vi "Pendant, show poses.vi"() -> (1 "position":string, 3 "group":string)   [LabVIEW 2013]
uses:
  <vilib>/Utility/config.llb/NI_LVConfig.lvlib
panel:
  in  "tab":T1(tab)
  in  "Groups":i32(listbox)
  in  "position":i32(listbox)
  in  "continue":bool
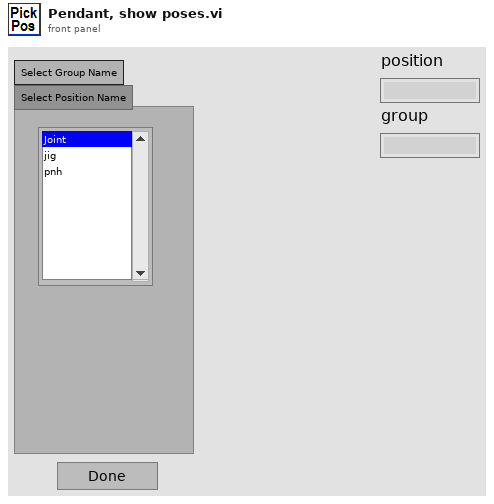
[diagram p1: front panel]
types:
  T1 = enum32{"Select Group Name", "Select Position Name"}
  T2 = typedef "NI_LVConfig.lvlib/Config Data RefNum.ctl" = refnum<k1>
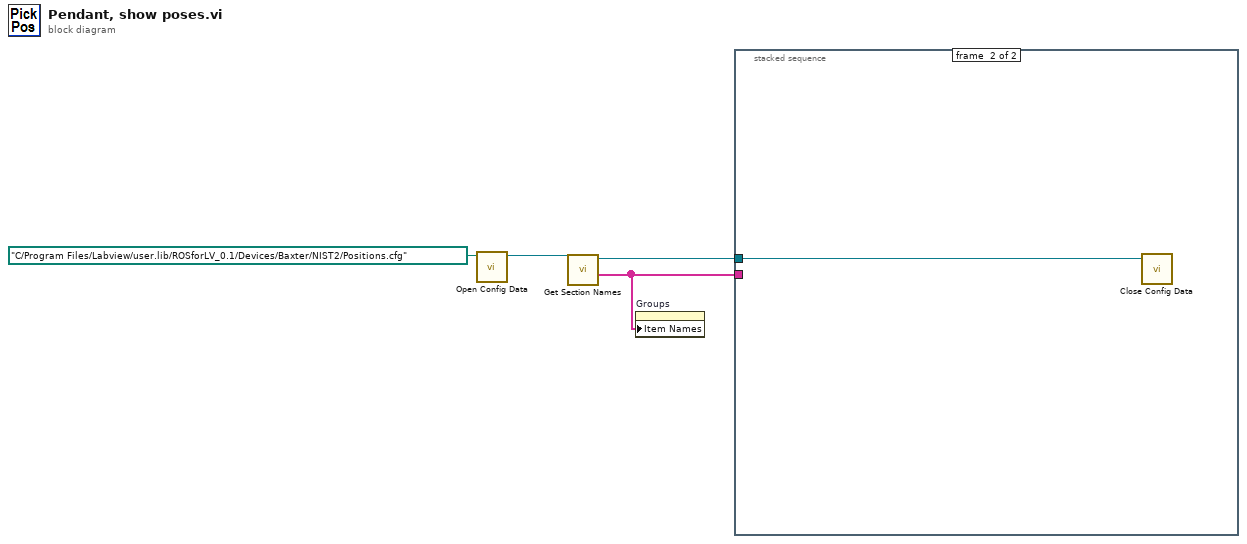
[diagram p0: block diagram]
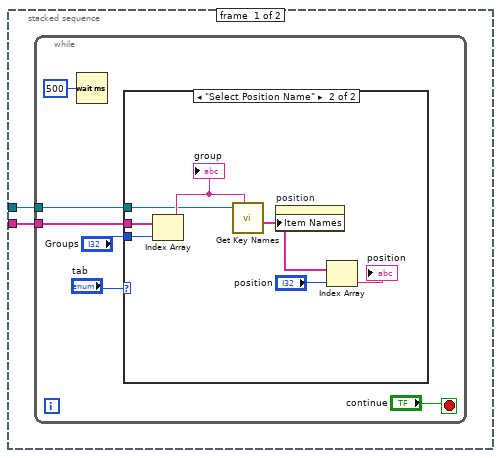
[diagram p2: hidden frame]
diagram:
  n1 = call <vilib>:"Open Config Data.vi"("configuration file path"=path "C:/Program Files/Labview/user.lib/ROSforLV_0.1/Devices/Baxter/NIST2/Positions.cfg") -> ("refnum"=w3:T2)  [unwired: 8 in, 2 out]
  n2 = call <vilib>:"Get Section Names.vi"("refnum"=w3) -> ("section names"=w2:string[], "refnum out"=w1:T2)  [unwired: 8 in, 1 out]
  n3 = property on="Groups" class="LstBox (strict)"("Item Names"=w2) -> ()  [unwired: 2 in, 2 out]
  n4 = stacked-sequence {
    tunnel: w2 -> [w6 _]
    tunnel: w1 -> [w5 w20]
    frame #0 {
      n5 = while {
        tunnel: w6 -> [w11]
        tunnel: w5 -> [w9]
        stop <- "continue" stop-if-true
        n6 = Wait (ms)(milliseconds to wait=u32 500) -> ()  [unwired: 1 out]
        n7 = case shown="\"Select Position Name\"" "tab" {
          tunnel: w11 -> [_ w19]
          tunnel: "Groups" -> [_ w18]
          tunnel: w9 -> [_ w16]
          frame "Select Group Name", Default {
          }
          frame "Select Position Name" {
            n8 = Index Array(array=w19, index=w18) -> (element=w17:string)
            "group" <- w17
            n9 = call <vilib>:"Get Key Names.vi"("section"=w17, "refnum"=w16) -> ("key names"=w15:string[])  [unwired: 6 in, 3 out]
            n10 = property on="position" class="LstBox (strict)"("Item Names"=w15) -> ()  [unwired: 2 in, 2 out]
            n11 = Index Array(array=w15, index="position") -> (element=→"position":string)
          }
        }
      }
    }
    frame #1 {
      n12 = call <vilib>:"Close Config Data.vi"("refnum"=w20) -> ()  [unwired: 9 in, 2 out]
    }
  }
